vi "Append Image to Report (path wrap).vi"(0 "report in":refnum<class "NI_report.lvclass">, 1 "alignment (default)":T1, 2 "MS Office parameters":T2, 7 "path or URL of image":path, 9 "caption or alternative string":string, 11 "error in (no error)":errorcluster) -> (4 "report out":refnum<class "NI_report.lvclass">, 6 "String":string, 8 "start out (Word)":i32, 10 "end out (Word)":i32, 15 "error out":errorcluster)   [LabVIEW 2013]
doc: "For an HTML report, the VI embeds a link to an image into the report. (Windows) For a standard report, the VI appends the image from a file. Standard reports support .bmp, .gif, .wmf, .emf, and .jpg image files. \n\nYou can wire either a path to the image or a string that contains the image URL to this polymorphic VI. Wire data to the <B>path or URL of image</B> input to determine the polymorphic instance to use or manually select the instance."
uses:
  <vilib>/Utility/NIReport.llb/NI_report.lvclass
  <vilib>/Utility/NIReport.llb/HTML Report Image Alignment.ctl
  <vilib>/Utility/NIReport.llb/NI_ReportGenerationCore.lvlib
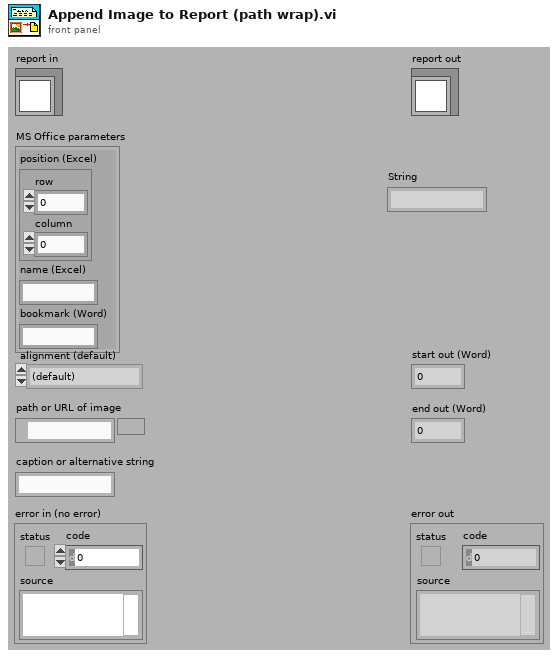
[diagram p1: front panel]
types:
  T1 = typedef "NI_ReportGenerationCore.lvlib/HTML Report Image Alignment.ctl" = enum16{"(default)", "LEFT", "RIGHT", "TOP", "TEXTTOP", "MIDDLE", "ABSMIDDLE", "BASELINE", "BOTTOM", "ABSBOTTOM"}
  T2 = cluster{"position (Excel)":cluster{"row":i32, "column":i32}, "name (Excel)":string, "bookmark (Word)":string}
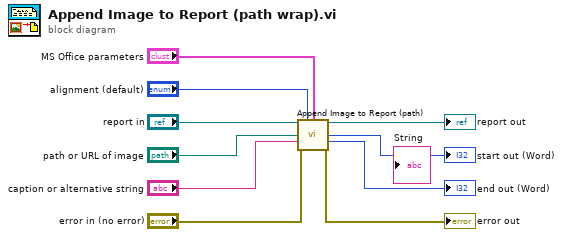
[diagram p0: block diagram]
diagram:
  n1 = call-dynamic "Append Image to Report (path).vi"("report in"="report in", "alignment (default)"="alignment (default)", "MS Office parameters"="MS Office parameters", "path or URL of image"="path or URL of image", "caption or alternative string"="caption or alternative string", "error in (no error)"="error in (no error)") -> ("report out"=→"report out":refnum<class "NI_report.lvclass">, "start out (Word)"=→"start out (Word)":i32, "end out (Word)"=→"end out (Word)":i32, "error out"=→"error out":errorcluster)  [unwired: 6 out]
